vi "Update Audio Analyzer Display Objects.vi"(8 "Error In":errorcluster, 11 "Display Manager In":refnum<class "Display Manager.lvclass">) -> (0 "Error Out":errorcluster, 3 "Display Manager Out":refnum<class "Display Manager.lvclass">)   [LabVIEW 2019, in "Display Manager.lvclass"]
uses:
  Display Manager.lvclass
  <vilib>/Memosfet/myRIO-Neopixel/RT/Graph/Graph.lvclass
  Accessors/Audio Spectrum Notifier/Get Audio Spectrum Notifier.vi
  Accessors/Display/Get Display.vi
  <vilib>/Memosfet/myRIO-Neopixel/RT/Display/Display.lvclass
  <vilib>/Memosfet/myRIO-Neopixel/RT/Display Element/Display Element.lvclass
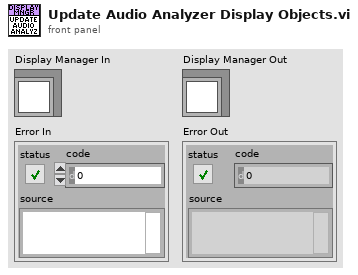
[diagram p1: front panel]
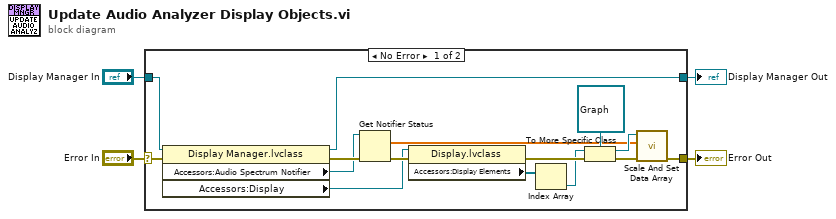
[diagram p0: block diagram]
diagram:
  n1 = case shown="No Error" "Error In" {
    selector: "Error In" -> [w18 w21]
    tunnel: [w8 w21] -> w3
    tunnel: "Display Manager In" -> [w19 w20]
    tunnel: [w17 w20] -> w1
    frame No Error {
      n2 = property class="Display Manager.lvclass"(reference=w19, error in=w18) -> (reference out=w17:refnum<class "Display Manager.lvclass">, error out=w10:errorcluster, "Accessors:Audio Spectrum Notifier"=w6:refnum<notifier>, "Accessors:Display"=w7:refnum<class "Display.lvclass">)
      n3 = Get Notifier Status(notifier=w6, error in (no error)=w10) -> (current notification=w5:dbl[], error out=w9:errorcluster)  [unwired: 3 out]
      n4 = property class="Display.lvclass"(reference=w7, error in=w9) -> (error out=w15:errorcluster, "Accessors:Display Elements"=w16:refnum<class "Display Element.lvclass">[])  [unwired: 1 out]
      n5 = Index Array(array=w16) -> (element=w13:refnum<class "Display Element.lvclass">)  [unwired: 1 in]
      n6 = To More Specific Class(target class=refnum<class "Graph.lvclass"> refnum ("Graph In"), reference=w13, error in=w15) -> (specific class reference=w12:refnum<class "Graph.lvclass">, error out=w11:errorcluster)
      n7 = call <vilib>:"Scale And Set Data Array.vi"("Error In"=w11, "Data Array"=w5, "Graph In"=w12) -> ("Error Out"=w8:errorcluster)  [unwired: 7 in, 1 out]
    }
    frame Error {
    }
  }
  "Display Manager Out" <- w1
  "Error Out" <- w3
